vi "正反控制.vi"(2 "接法":bool, 3 "x":dbl format="%#_13g") -> (0 "INB":bool, 1 "INA":bool)   [LabVIEW 2016]
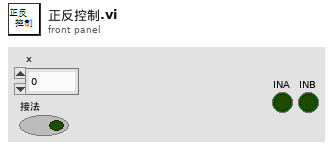
[diagram p1: front panel]
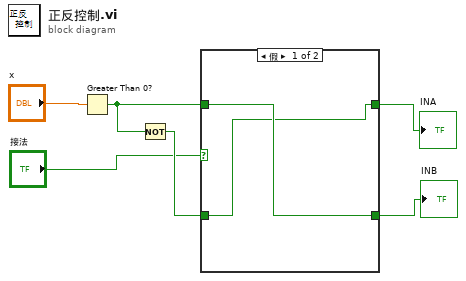
[diagram p0: block diagram]
diagram:
  n1 = Greater Than 0?(x="x") -> (x > 0?=w5:bool)
  n2 = Not(x=w5) -> (.not. x?=w4:bool)
  n3 = case shown="假" "接法" {
    tunnel: w5 -> [w8 w10]
    tunnel: w4 -> [w7 w9]
    tunnel: [w7 w10] -> w2
    tunnel: [w8 w9] -> w1
    frame False {
    }
    frame True {
    }
  }
  "INA" <- w2
  "INB" <- w1
